vi "HandleError.vi"(8 "error in (no error)":errorcluster, 11 "Source":string) -> (0 "error out":errorcluster)   [LabVIEW 2017, in "ErrorMonitor.lvlib"]
uses:
  ErrorMonitor.lvlib
  Queue/TypeDefs/queueFGVState.ctl
  Queue/TypeDefs/message.ctl
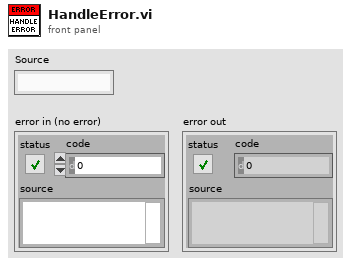
[diagram p1: front panel]
types:
  T1 = typedef "ErrorMonitor.lvlib/queueFGVState.ctl" = enum16{"obtain", "enqueue low priority", "enqueue high priority", "dequeue", "release"}
  T2 = typedef "ErrorMonitor.lvlib/message.ctl" = cluster{"calling module":string, "message":string, "Data":variant}
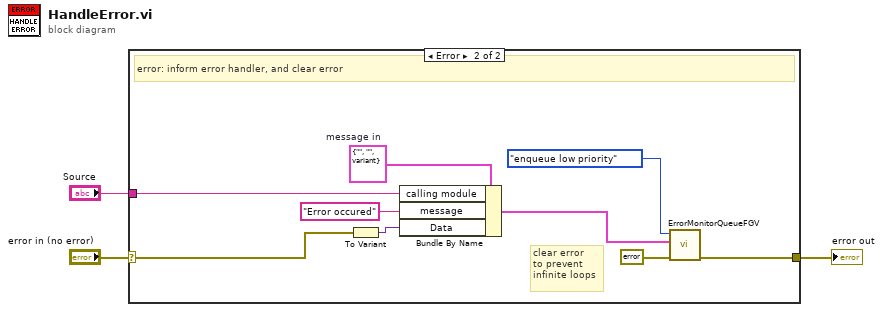
[diagram p0: block diagram]
diagram:
  n1 = case shown="Error" "error in (no error)" {
    selector: "error in (no error)" -> [w4 w8]
    tunnel: "Source" -> [_ w11]
    tunnel: [w4 w7] -> w1
    frame No Error {
      # "no error: do nothing"
    }
    frame Error {
      w12 = T2 {"calling module"="", "message"="", "Data"=variant}  # message in
      # "clear error\nto prevent\ninfinite loops"
      # "error: inform error handler, and clear error"
      n2 = To Variant(anything=w8) -> (Variant=w9:variant)
      n3 = Bundle By Name(cluster=w12, "calling module"=w11, "message"="Error occured", "Data"=w9) -> (w5:T2)
      n4 = call "ErrorMonitorQueueFGV.vi"("error in (no error)"=errorcluster {"status"=FALSE, "code"=0, "source"=""} ("error constant"), "message in"=w5, "Enum"=queueFGVState."enqueue low priority") -> ("error out"=w7:errorcluster)  [unwired: 7 in, 1 out]
    }
  }
  "error out" <- w1
